vi "wavelengh exporter.vi"() -> ()   [LabVIEW 2012]
uses:
  <vilib>/Utility/file.llb/Read From Spreadsheet File (DBL).vi
panel:
  in  "Time and wavelengh":dbl[](array[numeric])=[0.0, 260.0, 550.0, 647.0]
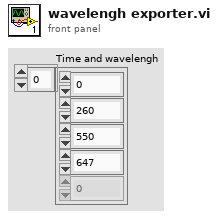
[diagram p1: front panel]
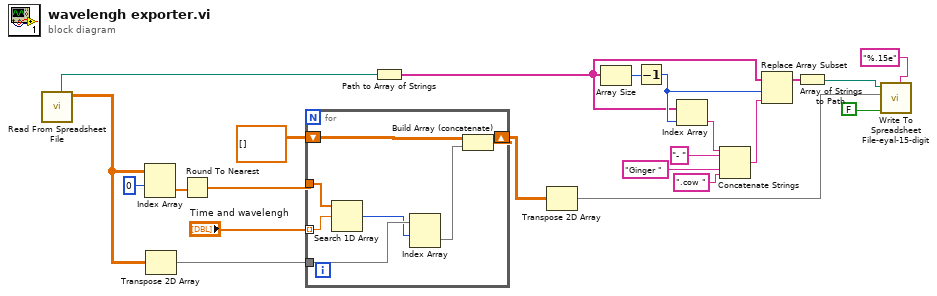
[diagram p0: block diagram]
diagram:
  n1 = call-poly <vilib>:"Read From Spreadsheet File.vi"() -> ("all rows"=w22:dbl[][], "new file path (Not A Path if cancelled)"=w4:path)  [unwired: 7 in, 3 out]
  n2 = Index Array(array=w22, index (row)=0) -> (element=w20:dbl[])  [unwired: 1 in]
  n3 = Transpose 2D Array(2D array=w22) -> (transposed array=w18:dbl[][])
  n4 = Round To Nearest(number=w20) -> (nearest integer value=w19:dbl[])
  n5 = for {
    tunnel: w19 -> [w29]
    tunnel: w18 -> [w28]
    tunnel: "Time and wavelengh" -> [w26] mode=indexing
    shift-right: [w25] -> w2
    shift-left: dbl[][] [] -> [w24]
    n6 = Search 1D Array(1D array=w29, element=w26) -> (index of element=w27:i32)  [unwired: 1 in]
    n7 = Index Array(array=w28, index (row)=w27) -> (element=w23:dbl[])  [unwired: 1 in]
    n8 = Build Array (concatenate)(w24, w23) -> (w25:dbl[][])
  }
  n9 = Path to Array of Strings(0:w4) -> (2:w9:string[])  [unwired: 1 out]
  n10 = Transpose 2D Array(2D array=w2) -> (transposed array=w1:dbl[][])
  n11 = Array Size(array=w9) -> (size(s)=w13:i32)
  n12 = Decrement(x=w13) -> (x-1=w11:i32)
  n13 = Index Array(array=w9, index=w11) -> (element=w12:string)
  n14 = Concatenate Strings(w12, "- " ("comand"), "Ginger " ("comand"), ".cow " ("comand")) -> (w10:string)
  n15 = Replace Array Subset(array=w9, new element=w10, index=w11) -> (w8:string[])
  n16 = Array of Strings to Path(0:w8) -> (2:w7:path)  [unwired: 1 in]
  n17 = call "Write To Spreadsheet File-eyal-15-digit.vi"("format (%.3f)"="%.15e", "append to file? (new file:F)"=FALSE, "2D data"=w1, "file path (dialog if empty)"=w7) -> ()  [unwired: 4 in, 1 out]
